vi "Create NI 9437 - Counter PWM Input.vi"(8 "error in":errorcluster, 10 "channel settings":T1[](array[typedef])) -> (0 "error out":errorcluster, 3 "NI 9437 out":refnum<class "NI 9437.lvclass">)   [LabVIEW 2017, in "Scan Engine Scripting.lvlib" / "NI 9437.lvclass"]
uses:
  NI 9437.lvclass
  Mode Classes/Controls/counter pwm input channel settings.ctl
  Channel Classes/PWM Input Channel/Measurement Type.ctl
  Mode Classes/Counter PWM Input Mode/Counter PWM Input Mode.lvclass
  C:/dev/github.com/debryant/niveristand-scan-engine-ethercat-custom-device/Custom Device Source/Scripting/Modules/Mode Classes/Mode/Mode.lvclass
  00c94b37-37fe-4450-80ce-a87fb43ff01e.vi
  Channel Classes/PWM Input Channel/PWM Input Channel.lvclass
  Scan Engine Scripting.lvlib
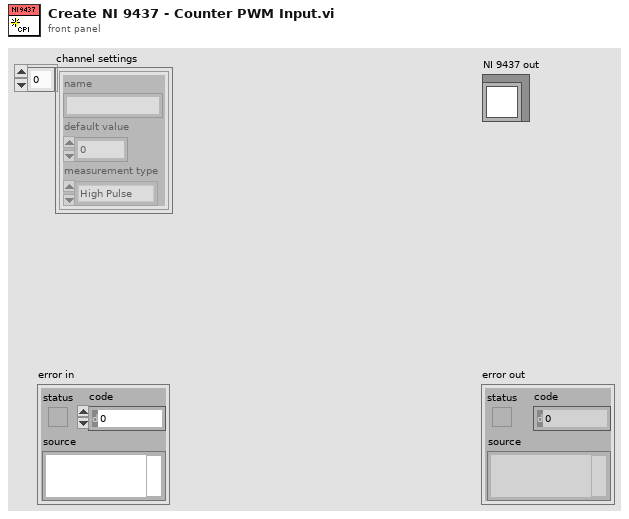
[diagram p1: front panel]
types:
  T1 = typedef "Scan Engine Scripting.lvlib/counter pwm input channel settings.ctl" = cluster{"name":string, "default value":dbl, "measurement type":T2}
  T2 = typedef "Scan Engine Scripting.lvlib/PWM Input Channel.lvclass/Measurement Type.ctl" = enum16{"High Pulse", "Low Pulse", "Most Recent"}
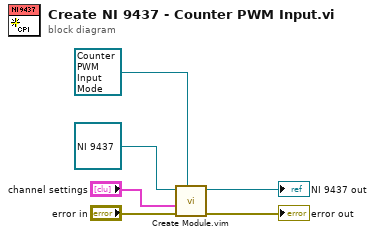
[diagram p0: block diagram]
diagram:
  n1 = call "Create Module.vim"("mode in"=refnum<class "Counter PWM Input Mode.lvclass"> refnum ("Scan Engine Scripting.lvlib:Counter PWM Input Mode.lvclass"), "error in"="error in", "channel settings"="channel settings", "module in"=refnum<class "NI 9437.lvclass"> refnum ("Scan Engine Scripting.lvlib:NI 9437.lvclass")) -> ("error out"=→"error out":errorcluster, "module out"=→"NI 9437 out":refnum<class "NI 9437.lvclass">)  [unwired: 6 in]
